vi "Launcher.vi"   [LabVIEW 2024, in "App.lvclass"]
uses:
  App.lvclass
  GUI/View/View.lvclass
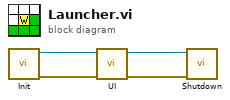
[diagram p0: block diagram]
diagram:
  n1 = call "Init.vi"() -> ("error out"=w2:errorcluster, "View out"=w4:refnum<class "View.lvclass">)  [unwired: 10 in]
  n2 = call "UI.vi"("error in (no error)"=w2, "View in"=w4) -> ("error out"=w1:errorcluster, "View out"=w3:refnum<class "View.lvclass">)  [unwired: 8 in]
  n3 = call "Shutdown.vi"("error in (no error)"=w1, "View in"=w3) -> ()  [unwired: 8 in, 2 out]
